vi "NET_Enable_System.vi"(4 "Read(F) Write(T)":bool, 5 "Enable RIO In":bool, 6 "Enable PCM In":bool, 7 "Enable PDP In":bool) -> (1 "Enable RIO Out":bool, 2 "Enable PCM Out":bool, 3 "Enable PDP Out":bool)   [LabVIEW 2017]
uses:
  <vilib>/Rock Robotics/Network Tables/NT Read Boolean Array.vi
  <vilib>/Rock Robotics/Network Tables/NT Write Boolean Array.vi
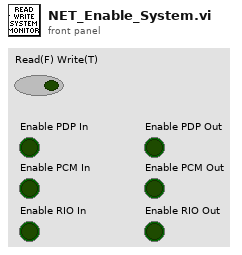
[diagram p1: front panel]
types:
  T1 = cluster{"Enable PDP In":bool, "Enable RIO In":bool, "Enable PCM In":bool}
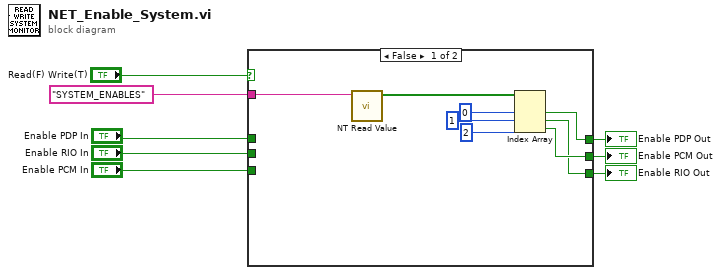
[diagram p0: block diagram]
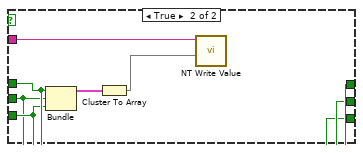
[diagram p2: hidden frame]
diagram:
  n1 = case shown="False" "Read(F) Write(T)" {
    tunnel: "SYSTEM_ENABLES" ("Name") -> [w16 w22]
    tunnel: "Enable PDP In" -> [_ w19]
    tunnel: "Enable RIO In" -> [_ w17]
    tunnel: "Enable PCM In" -> [_ w18]
    tunnel: [w11 w19] -> w3
    tunnel: [w10 w18] -> w2
    tunnel: [w9 w17] -> w1
    frame False {
      n2 = call-poly <vilib>:"NT Read Value.vi"("Name"=w16) -> ("Boolean Array"=w15:bool[])  [unwired: 9 in, 1 out]
      n3 = Index Array(array=w15, index #1=0 ("index"), index #2=1 ("index"), index #3=2 ("index")) -> (element #1=w11:bool, element #2=w9:bool, element #3=w10:bool)
    }
    frame True {
      n4 = Bundle("Enable PDP In"=w19, "Enable RIO In"=w17, "Enable PCM In"=w18) -> (w21:T1)  [unwired: 1 in]
      n5 = Cluster To Array(cluster=w21) -> (array=w20:bool[])
      n6 = call-poly <vilib>:"NT Write Value.vi"("Boolean Array"=w20, "Name"=w22) -> ()  [unwired: 9 in, 1 out]
    }
  }
  "Enable PCM Out" <- w2
  "Enable PDP Out" <- w3
  "Enable RIO Out" <- w1
